vi "BuildMaxHeap.vi"(8 "Error in (no error)":errorcluster, 11 "Heap in":refnum<class "UintClass.lvclass">[](array[class])) -> (0 "Error out":errorcluster, 3 "Heap out":refnum<class "UintClass.lvclass">[](array[class]))   [LabVIEW 2011, in "UintClass.lvclass"]
uses:
  UintClass.lvclass
  uintGreater.vi
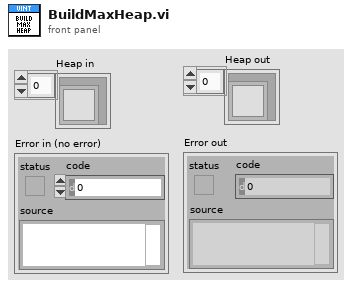
[diagram p1: front panel]
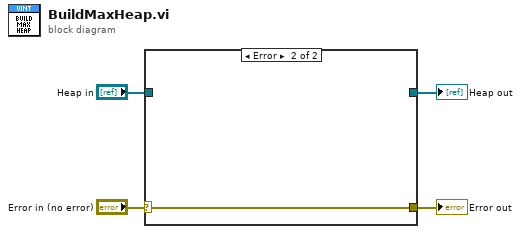
[diagram p0: block diagram]
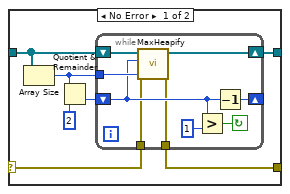
[diagram p2: hidden frame]
diagram:
  n1 = case shown="Error" "Error in (no error)" {
    selector: "Error in (no error)" -> [w5 w21]
    tunnel: "Heap in" -> [w11 _]
    tunnel: [w10 _] -> w3
    tunnel: [w6 w21] -> w2
    frame No Error {
      n2 = Array Size(array=w11) -> (size(s)=w8:i32)
      n3 = Quotient & Remainder(x=w8, y=2) -> (floor(x/y)=w7:i32)  [unwired: 1 out]
      n4 = while {
        shift-right: [w20] -> _
        shift-left: w7 -> [w14]
        shift-right: [w18] -> w10
        shift-left: w11 -> [w19]
        tunnel: w8 -> [w15]
        tunnel: w5 -> [w13]
        tunnel: [w12] -> w6
        stop <- w16 continue-if-true
        n5 = call "MaxHeapify.vi"("Error in (no error)"=w13, "Length"=w15, "i"=w14, "Heap in"=w19) -> ("Error out"=w12:errorcluster, "Heap out"=w18:refnum<class "UintClass.lvclass">[])  [unwired: 6 in]
        n6 = Greater?(x=w14, y=1) -> (0:w16:bool)
        n7 = Decrement(x=w14) -> (x-1=w20:i32)
      }
    }
    frame Error {
    }
  }
  "Heap out" <- w3
  "Error out" <- w2
